vi "Store Parameters.vi"(8 "error in":errorcluster, 11 "PPT in":refnum<class "PPT.lvclass">) -> (0 "error out":errorcluster, 3 "PPT out":refnum<class "PPT.lvclass">)   [LabVIEW 2014, in "PPT Library.lvlib" / "PPT.lvclass"]
doc: "Store all current parameters in RAM to EEPROM (where applicable)."
uses:
  PPT.lvclass
  reusable/Session APIs/Serial/Serial Session.lvclass
  PPT.lvclass/PPT.ctl
  Accessors/Read Address.vi
  Accessors/Read Serial Session.vi
  reusable/Session APIs/Serial/Public/Asynchronous Write.vi
  <userlib>/_Session Fwk/Session - Root.lvclass
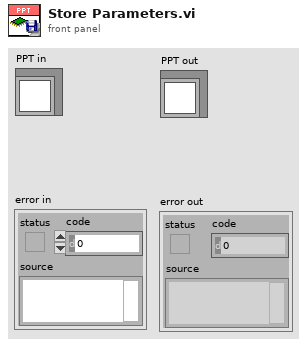
[diagram p1: front panel]
types:
  T1 = typedef "Session - Root.lvclass/Session Handle.ctl" = refnum<data-value>
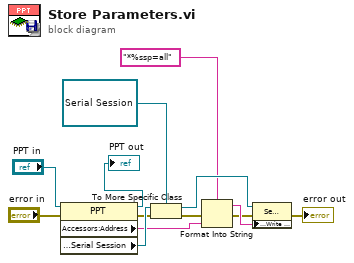
[diagram p0: block diagram]
diagram:
  n1 = property class="PPT"(reference="PPT in", error in="error in") -> (reference out=→"PPT out":refnum<class "PPT.lvclass">, error out=w5:errorcluster, "Accessors:Address"=w7:string, "Accessors:Serial Session"=w8:T1)
  n2 = To More Specific Class(target class=refnum<data-value> refnum, reference=w8, error in=w5) -> (specific class reference=w13:refnum<data-value>, error out=w11:errorcluster)
  n3 = Format Into String(format string="*%ssp=all", error in=w11, w7) -> (resulting string=w12:string, error out=w10:errorcluster)  [unwired: 1 in]
  n4 = property class="Serial Session"(reference=w13, error in=w10, "Public:Write - Asynchronous"=w12) -> (error out=→"error out":errorcluster)  [unwired: 1 out]
